vi "Acquire Class Details_Get Member VIs.vi"(7 "Dynamic dispatch?":bool, 8 "error in (no error)":errorcluster, 10 "Class Path":path, 11 "Member VIs (auto closed)":refnum<vi>[](array[refnum])) -> (0 "error out":errorcluster, 3 "Member Array":T1[](array[typedef]))   [LabVIEW 2020, in "ClassLoader.lvlib"]
uses:
  ClassLoader.lvlib
  <vilib>/Utility/Data Type/Member VI Info.ctl
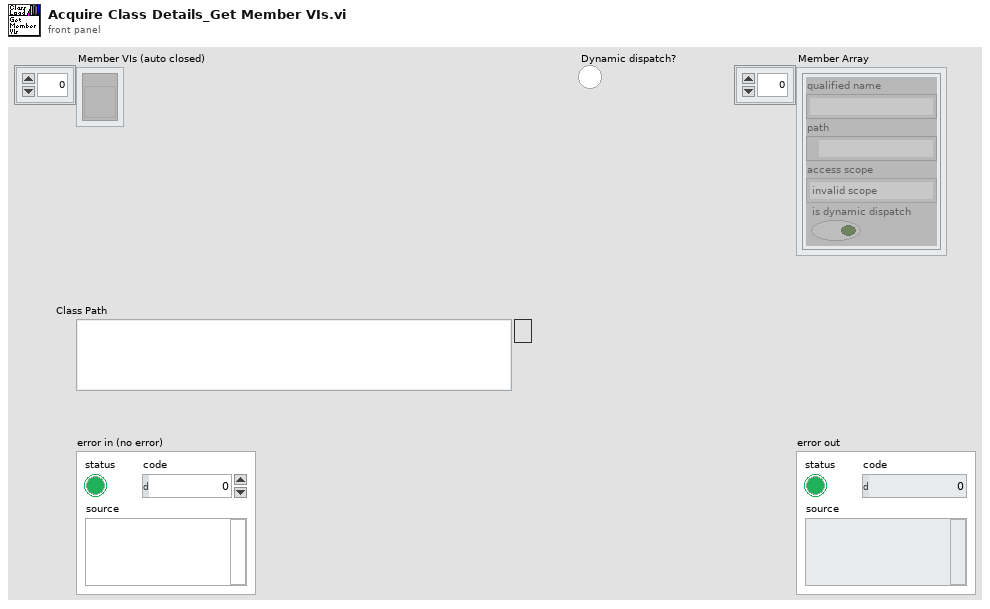
[diagram p1: front panel]
types:
  T1 = typedef "Member VI Info.ctl" = cluster{"qualified name":string, "path":path, "access scope":enum32{"invalid scope", "public", "private", "protected", "community"}, "is dynamic dispatch":bool}
  T2 = enum32{"invalid scope", "public", "private", "protected", "community"}
  T3 = enum32{"invalid scope", "public", "private", "protected", "community"}[]
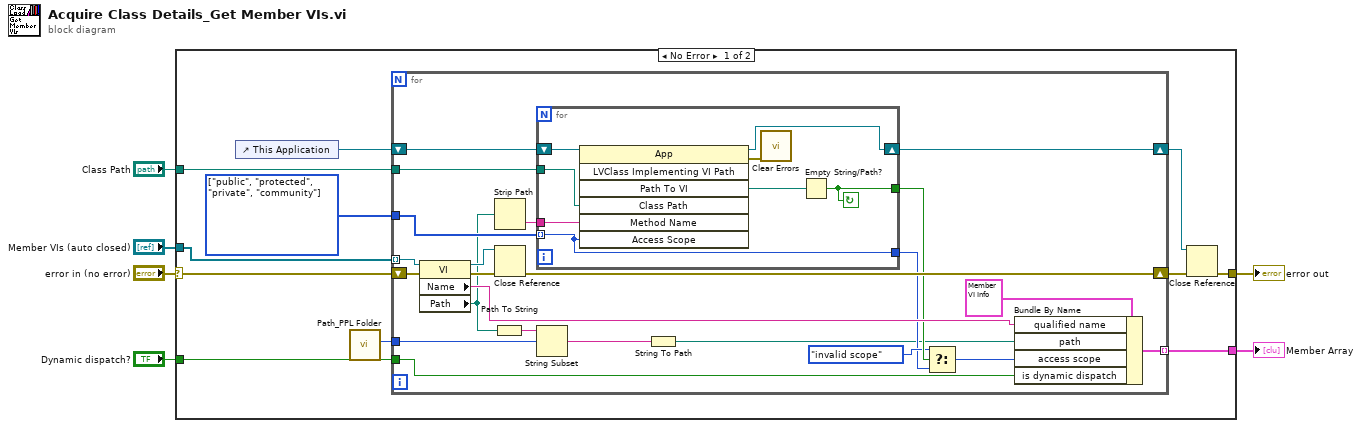
[diagram p0: block diagram]
diagram:
  n1 = case shown="No Error" "error in (no error)" {
    selector: "error in (no error)" -> [w16 w49]
    tunnel: "Dynamic dispatch?" -> [w17 _]
    tunnel: [w15 _] -> w4
    tunnel: "Member VIs (auto closed)" -> [w14 _]
    tunnel: [w10 w49] -> w2
    tunnel: "Class Path" -> [w9 _]
    frame No Error {
      w8 = T3 [enum."public", enum."protected", enum."private", enum."community"] items=["invalid scope", "public", "private", "protected", "community"] ("Access Scope")
      n2 = control-ref of="This Application"() -> (w13:refnum<vi>)
      n3 = call "Path_PPL Folder.vi"() -> ("Path Length"=w7:i32)  [unwired: 10 in, 1 out]
      n4 = for {
        tunnel: w14 -> [w40] mode=indexing
        tunnel: [w38] -> w15 mode=indexing
        shift-right: [w36] -> w11
        shift-left: w16 -> [w37]
        tunnel: w17 -> [w35]
        shift-right: [w29] -> w12
        shift-left: w13 -> [w33]
        tunnel: w9 -> [w32]
        tunnel: w8 -> [w30]
        tunnel: w7 -> [w20]
        n5 = property class="VI"(reference=w40, error in=w37) -> (reference out=w39:refnum<vi>, error out=w34:errorcluster, "Name"=w31:string, "Path"=w22:path)
        n6 = Path To String(path=w22) -> (string=w21:string)
        n7 = Strip Path(path=w22) -> (name=w24:string)  [unwired: 1 out]
        n8 = Close Reference(reference=w39, error in (no error)=w34) -> (error out=w36:errorcluster)
        n9 = for {
          tunnel: w32 -> [w47]
          tunnel: w24 -> [w46]
          tunnel: w30 -> [w44] mode=indexing
          shift-right: [w45] -> w29
          shift-left: w33 -> [w48]
          tunnel: [w42] -> w28
          tunnel: [w44] -> w26
          stop <- w42 continue-if-true
          n10 = invoke class="App" method="LVClass Implementing VI Path"(reference=w48, "Class Path"=w47, "Method Name"=w46, "Access Scope"=w44) -> (reference out=w45:refnum<vi>, error out=w41:errorcluster, "Path To VI"=w43:path)  [unwired: 3 in, 4 out]
          n11 = call <vilib>:"Clear Errors.vi"("error in (no error)"=w41) -> ()  [unwired: 5 in, 2 out]
          n12 = Empty String/Path?(string/path=w43) -> (empty?=w42:bool)
        }
        n13 = String Subset(string=w21, offset (0)=w20) -> (substring=w19:string)  [unwired: 1 in]
        n14 = String To Path(string=w19) -> (path=w18:path)
        n15 = Select(t=T2."invalid scope" ("Access Scope"), s=w28, f=w26) -> (s? t:f=w25:T2)
        n16 = Bundle By Name(cluster=T1 {"qualified name"="", "path"=path "", "access scope"=enum."invalid scope", "is dynamic dispatch"=FALSE} ("VI info"), "qualified name"=w31, "path"=w18, "access scope"=w25, "is dynamic dispatch"=w35) -> (w38:T1)
      }
      n17 = Close Reference(reference=w12, error in (no error)=w11) -> (error out=w10:errorcluster)
    }
    frame Error {
    }
  }
  "error out" <- w2
  "Member Array" <- w4
